vi "Traffic Lights Visualisation.vi"() -> ()   [LabVIEW 2018]
uses:
  Lights Display.ctl
  Color states.ctl
  <vilib>/lvdsc/NI_DSC.lvlib
panel:
  in  "Background":u32(colorbox)=9079434
  out "Color time 3":i32
  out "Color time 4":i32
  out "Color time 1":i32 format="%.0p"
  out "Color time 2":i32
  in  "Time scale":dbl
  out "Simulation Time":timestamp
  out "Traffic Lights 4":T1
  out "Traffic Lights 3":T1
  in  "Close window":bool
  in  "Showsettings":bool
  out "Traffic Lights 2":T1
  out "Traffic Lights 1":T1
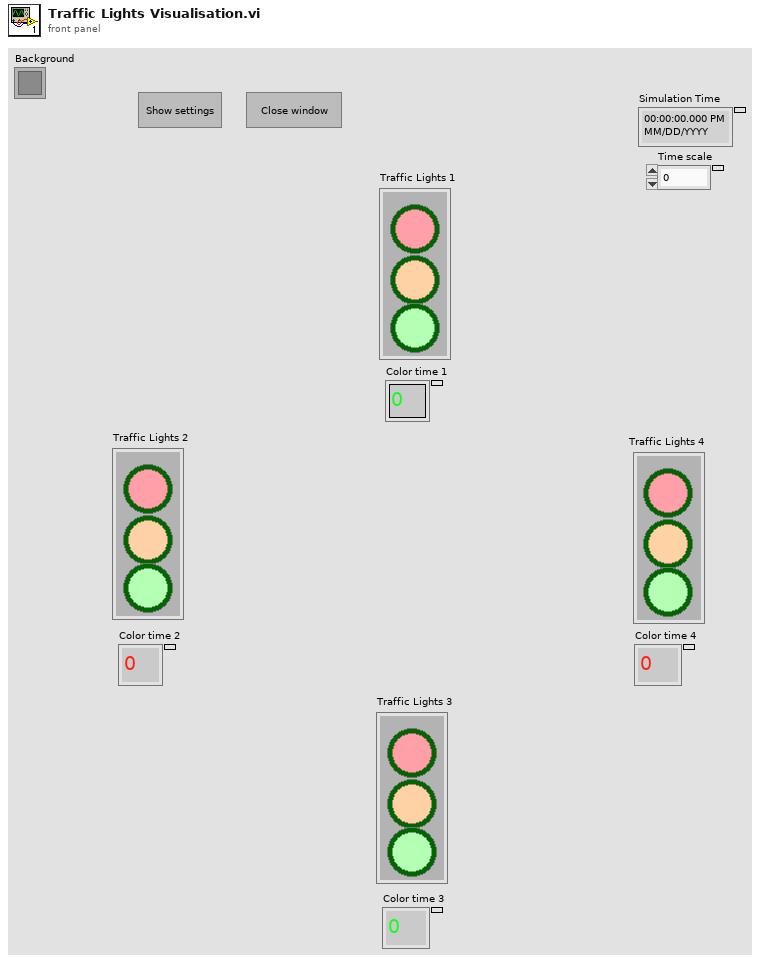
[diagram p1: front panel]
types:
  T1 = typedef "Lights Display.ctl" = cluster{"Red":bool, "Amber":bool, "Green":bool}
  T2 = typedef "Color states.ctl" = enum16{"Green", "Red-Yellow", "Yellow", "Red", "Null"}
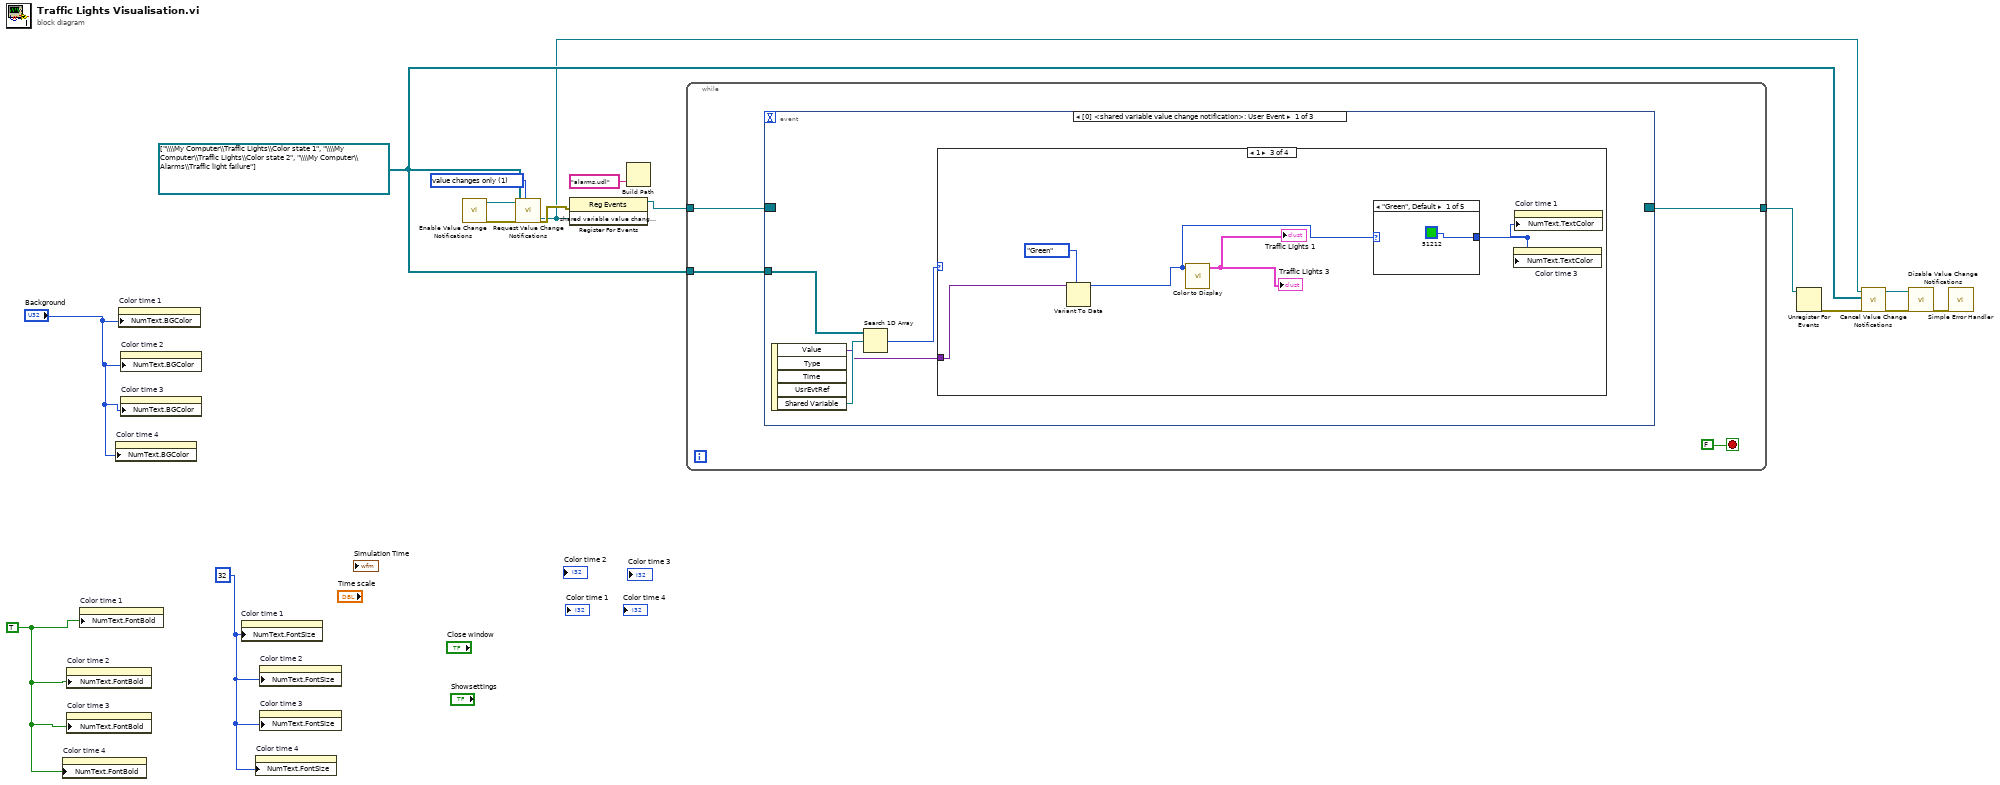
[diagram p0: block diagram]
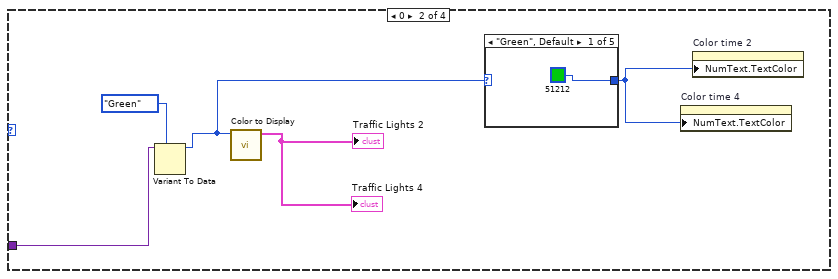
[diagram p3: hidden frame]
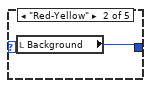
[diagram p4: hidden frame]
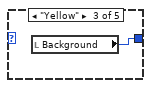
[diagram p5: hidden frame]
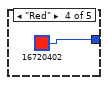
[diagram p6: hidden frame]
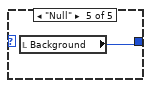
[diagram p7: hidden frame]
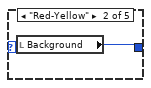
[diagram p8: hidden frame]
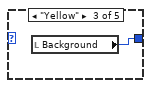
[diagram p9: hidden frame]
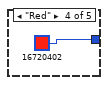
[diagram p10: hidden frame]
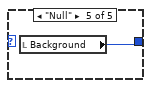
[diagram p11: hidden frame]
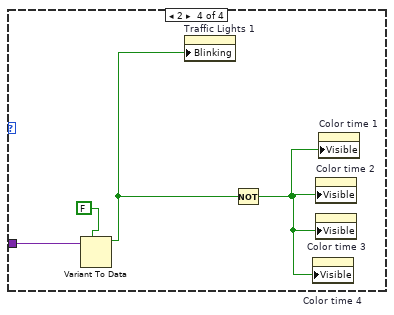
[diagram p12: hidden frame]
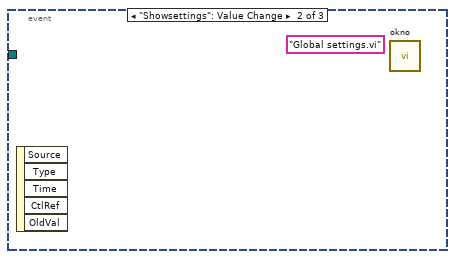
[diagram p13: hidden frame]
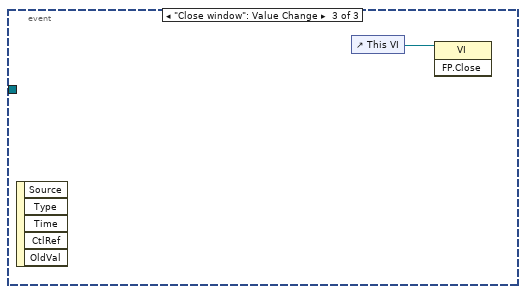
[diagram p14: hidden frame]
diagram:
  w2 = u32 32 ("Numeric Text.Size:Height")
  w3 = TRUE ("Numeric Text.Font:Bold")
  w5 = refnum<k21>[] ["\\\\My Computer\\Traffic Lights\\Color state 1", "\\\\My Computer\\Traffic Lights\\Color state 2", "\\\\My Computer\\Alarms\\Traffic light failure"] ("shared variables")
  w13 = u16 1 items=["all changes", "value changes only"] ("request changes (all changes)")
  n1 = property on="Color time 4" class="DigNum (strict)"("NumText.FontBold"=w3) -> ()  [unwired: 2 in, 2 out]
  n2 = property on="Color time 2" class="DigNum (strict)"("NumText.FontBold"=w3) -> ()  [unwired: 2 in, 2 out]
  n3 = property on="Color time 3" class="DigNum (strict)"("NumText.FontBold"=w3) -> ()  [unwired: 2 in, 2 out]
  n4 = property on="Color time 1" class="DigNum (strict)"("NumText.FontBold"=w3) -> ()  [unwired: 2 in, 2 out]
  n5 = property on="Color time 4" class="DigNum (strict)"("NumText.BGColor"="Background") -> ()  [unwired: 2 in, 2 out]
  n6 = property on="Color time 1" class="DigNum (strict)"("NumText.BGColor"="Background") -> ()  [unwired: 2 in, 2 out]
  n7 = property on="Color time 2" class="DigNum (strict)"("NumText.BGColor"="Background") -> ()  [unwired: 2 in, 2 out]
  n8 = property on="Color time 3" class="DigNum (strict)"("NumText.BGColor"="Background") -> ()  [unwired: 2 in, 2 out]
  n9 = property on="Color time 1" class="DigNum (strict)"("NumText.FontSize"=w2) -> ()  [unwired: 2 in, 2 out]
  n10 = property on="Color time 4" class="DigNum (strict)"("NumText.FontSize"=w2) -> ()  [unwired: 2 in, 2 out]
  n11 = property on="Color time 2" class="DigNum (strict)"("NumText.FontSize"=w2) -> ()  [unwired: 2 in, 2 out]
  n12 = property on="Color time 3" class="DigNum (strict)"("NumText.FontSize"=w2) -> ()  [unwired: 2 in, 2 out]
  n13 = call <vilib>:"Enable Value Change Notifications.vi"() -> ("error out"=w16:errorcluster, "shared variable value change notification"=w15:refnum<user-event>)  [unwired: 1 in, 9 out]
  n14 = call <vilib>:"Request Value Change Notifications.vi"("request changes (all changes)"=w13, "error in (no error)"=w16, "shared variables"=w5, "notification refnum"=w15) -> ("error out"=w14:errorcluster, "shared variable value change notification"=w4:refnum<user-event>)  [unwired: 6 out]
  n15 = register-events(error in=w14, w4) -> (reference out=w11:refnum<event-registration>)  [unwired: 1 in, 1 out]
  n16 = Build Path(name or relative path="alarms.udl") -> ()  [unwired: 1 in, 1 out]
  n17 = while {
    tunnel: w11 -> [w19]
    tunnel: w5 -> [w18]
    tunnel: [w17] -> w6
    stop <- FALSE stop-if-true
    n18 = event shown="[0] <shared variable value change notification>: User Event" {
      selector: w19 -> [_ _ _]
      dyn-events: [_ _ _] -> w17
      timeout: _ -> [_ _ _]
      tunnel: w18 -> [w24 _ _]
      event User Event {
        n19 = event-data() -> ("Value"=w21:variant, "Shared Variable"=w23:refnum<k21>)  [unwired: 1 in, 3 out]
        n20 = Search 1D Array(1D array=w24, element=w23) -> (index of element=w22:i32)  [unwired: 1 out]
        n21 = case shown="1" w22 {
          tunnel: w21 -> [_ w28 w38 w48]
          frame -1, Default {
          }
          frame 0 {
            n22 = Variant To Data(type=Color_states."Green" ("Color state 1"), Variant=w28) -> (data=w25:T2)  [unwired: 1 in, 1 out]
            n23 = call "Color to Display.vi"("Color state"=w25) -> ("Traffic Lights"=→"Traffic Lights 2" →"Traffic Lights 4":T1)  [unwired: 10 in]
            n24 = case shown="\"Green\", Default" w25 {
              tunnel: [u32 51212 w31 w32 u32 16720402 w34] -> w26
              frame "Green", Default {
              }
              frame "Red-Yellow" {
                n25 = local read "Background"() -> (w31:u32)
              }
              frame "Yellow" {
                n26 = local read "Background"() -> (w32:u32)
              }
              frame "Red" {
              }
              frame "Null" {
                n27 = local read "Background"() -> (w34:u32)
              }
            }
            n28 = property on="Color time 4" class="DigNum (strict)"("NumText.TextColor"=w26) -> ()  [unwired: 2 in, 2 out]
            n29 = property on="Color time 2" class="DigNum (strict)"("NumText.TextColor"=w26) -> ()  [unwired: 2 in, 2 out]
          }
          frame 1 {
            n30 = Variant To Data(type=Color_states."Green" ("Color state 1"), Variant=w38) -> (data=w36:T2)  [unwired: 1 in, 1 out]
            n31 = call "Color to Display.vi"("Color state"=w36) -> ("Traffic Lights"=→"Traffic Lights 1" →"Traffic Lights 3":T1)  [unwired: 10 in]
            n32 = case shown="\"Green\", Default" w36 {
              tunnel: [u32 51212 w41 w42 u32 16720402 w44] -> w35
              frame "Green", Default {
              }
              frame "Red-Yellow" {
                n33 = local read "Background"() -> (w41:u32)
              }
              frame "Yellow" {
                n34 = local read "Background"() -> (w42:u32)
              }
              frame "Red" {
              }
              frame "Null" {
                n35 = local read "Background"() -> (w44:u32)
              }
            }
            n36 = property on="Color time 3" class="DigNum (strict)"("NumText.TextColor"=w35) -> ()  [unwired: 2 in, 2 out]
            n37 = property on="Color time 1" class="DigNum (strict)"("NumText.TextColor"=w35) -> ()  [unwired: 2 in, 2 out]
          }
          frame 2 {
            n38 = Variant To Data(type=FALSE ("Blinking"), Variant=w48) -> (data=w46:bool)  [unwired: 1 in, 1 out]
            n39 = property on="Traffic Lights 1" class="Clust (strict)"("Blinking"=w46) -> ()  [unwired: 2 in, 2 out]
            n40 = Not(x=w46) -> (.not. x?=w45:bool)
            n41 = property on="Color time 4" class="DigNum (strict)"("Visible"=w45) -> ()  [unwired: 2 in, 2 out]
            n42 = property on="Color time 2" class="DigNum (strict)"("Visible"=w45) -> ()  [unwired: 2 in, 2 out]
            n43 = property on="Color time 3" class="DigNum (strict)"("Visible"=w45) -> ()  [unwired: 2 in, 2 out]
            n44 = property on="Color time 1" class="DigNum (strict)"("Visible"=w45) -> ()  [unwired: 2 in, 2 out]
          }
        }
      }
      event "Showsettings": Value Change {
        (unwired) "Global settings.vi" ("name or relative path")
        n45 = event-data() -> ()  [unwired: 1 in, 5 out]
        n46 = call "okno.vi"() -> ()  [unwired: 12 in]
      }
      event "Close window": Value Change {
        n47 = event-data() -> ()  [unwired: 1 in, 5 out]
        n48 = control-ref of="This VI"() -> (w49:refnum<vi>)
        n49 = invoke class="VI" method="FP.Close"(reference=w49) -> ()  [unwired: 2 in, 3 out]
      }
    }
  }
  n50 = Unregister For Events(event registration refnum=w6) -> (error out=w10:errorcluster)  [unwired: 1 in]
  n51 = call <vilib>:"Cancel Value Change Notifications.vi"("error in (no error)"=w10, "shared variables"=w5, "notification refnum"=w4) -> ("error out"=w9:errorcluster, "shared variable value change notification"=w8:refnum<user-event>)  [unwired: 7 out]
  n52 = call <vilib>:"Disable Value Change Notifications.vi"("error in (no error)"=w9, "notification refnum"=w8) -> ("error out"=w7:errorcluster)  [unwired: 9 out]
  n53 = call <vilib>:"Simple Error Handler.vi"("error in (no error)"=w7) -> ()  [unwired: 1 in, 8 out]
